vi "INDEX - Tree Control.vi"() -> ()   [LabVIEW 2011, in "VITesterUtilities.lvlib"]
uses:
  Libraries/VITesterUtilities.lvlib
panel:
  in  "Tree":string(tree)
  # "SEE BLOCK DIAGRAM FOR INDEX"
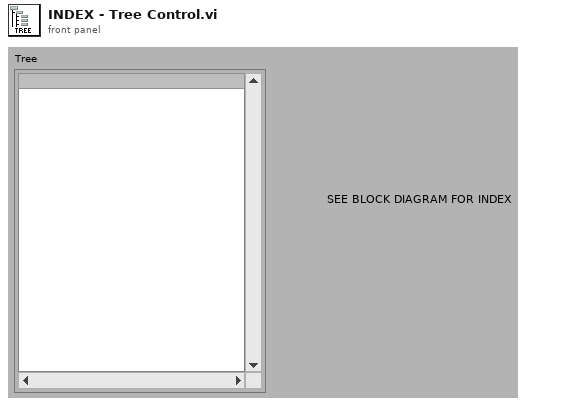
[diagram p1: front panel]
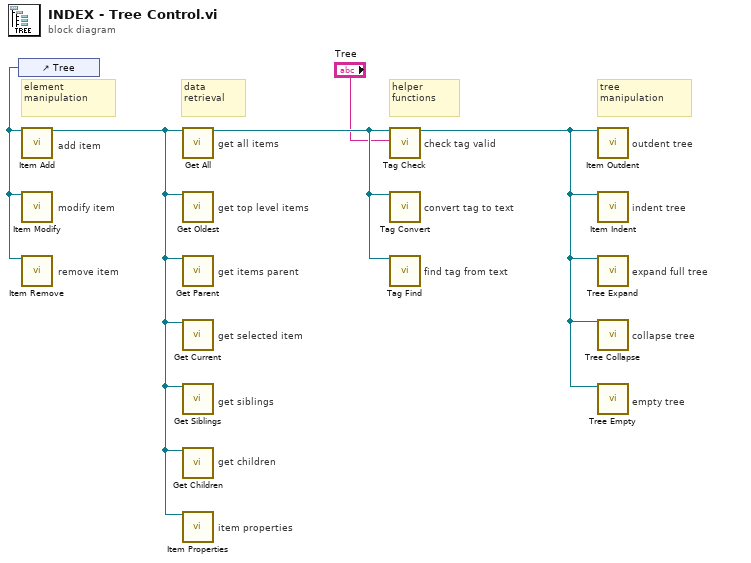
[diagram p0: block diagram]
diagram:
  # "empty tree"
  # "collapse tree"
  # "expand full tree"
  # "indent tree"
  # "outdent tree"
  # "find tag from text"
  # "convert tag to text"
  # "check tag valid"
  # "get children"
  # "get siblings"
  # "get selected item"
  # "get items parent"
  # "get top level items"
  # "get all items"
  # "item properties"
  # "remove item"
  # "modify item"
  # "add item"
  # "tree\nmanipulation"
  # "helper\nfunctions"
  # "data\nretrieval"
  # "element\nmanipulation"
  n1 = control-ref of="Tree"() -> (w2:refnum<vi>)
  n2 = call "Item Add.vi"("Tree Reference In"=w2) -> ("Tree Reference Out"=w3:refnum<vi>)  [unwired: 16 in, 2 out]
  n3 = call "Item Modify.vi"("Tree Reference In"=w2) -> ()  [unwired: 17 in, 2 out]
  n4 = call "Item Remove.vi"("Tree Reference In"=w2) -> ()  [unwired: 17 in, 2 out]
  n5 = call "Get All.vi"("Tree Reference In"=w3) -> ("Tree Reference Out"=w4:refnum<vi>)  [unwired: 15 in, 3 out]
  n6 = call "Get Oldest.vi"("Tree Reference In"=w3) -> ()  [unwired: 16 in, 3 out]
  n7 = call "Get Parent.vi"("Tree Reference In"=w3) -> ()  [unwired: 15 in, 4 out]
  n8 = call "Get Current.vi"("Tree Reference In"=w3) -> ()  [unwired: 15 in, 4 out]
  n9 = call "Get Siblings.vi"("Tree Reference In"=w3) -> ()  [unwired: 16 in, 3 out]
  n10 = call "Get Children.vi"("Tree Reference In"=w3) -> ()  [unwired: 16 in, 3 out]
  n11 = call "Item Properties.vi"("Tree Reference In"=w3) -> ()  [unwired: 13 in, 6 out]
  n12 = call "Tag Check.vi"("Tree Reference In"=w4, "Input Tag"="Tree") -> ("Tree Reference Out"=w5:refnum<vi>)  [unwired: 14 in, 3 out]
  n13 = call "Tag Convert.vi"("Tree Reference In"=w4) -> ()  [unwired: 15 in, 4 out]
  n14 = call "Tag Find.vi"("Tree Reference In"=w4) -> ()  [unwired: 15 in, 4 out]
  n15 = call "Item Outdent.vi"("Tree Reference In"=w5) -> ()  [unwired: 17 in, 2 out]
  n16 = call "Item Indent.vi"("Tree Reference In"=w5) -> ()  [unwired: 17 in, 2 out]
  n17 = call "Tree Expand.vi"("Tree Reference In"=w5) -> ()  [unwired: 17 in, 2 out]
  n18 = call "Tree Collapse.vi"("Tree Reference In"=w5) -> ()  [unwired: 17 in, 2 out]
  n19 = call "Tree Empty.vi"("Tree Reference In"=w5) -> ()  [unwired: 16 in, 3 out]
